vi "Configure Pattern Source.vi"(0 "VISA resource name":refnum<visa-resource-name>, 1 "Lower Threshold (1)":dbl, 2 "Data Mode (1: Fixed)":i32(ring) items=["Automatic", "Fixed"], 5 "Pattern Source (0: Internal)":i32(ring) items=["Internal", "External"], 7 "Voltage Range (5)":dbl, 9 "Impedance (1: 10000 Ohm)":i32(ring) items=["50 Ohm", "10000 Ohm"], 11 "error in (no error)":errorcluster, 12 "Upper Threshold (1.6)":dbl) -> (4 "VISA resource name out":refnum<visa-resource-name>, 15 "error out":errorcluster)   [LabVIEW 2009, in "Agilent 81150.lvlib"]
doc: "Configures the pattern source."
uses:
  Agilent 81150.lvlib
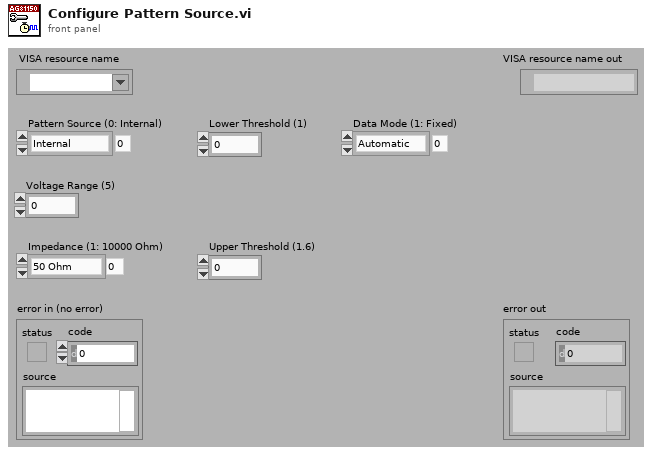
[diagram p1: front panel]
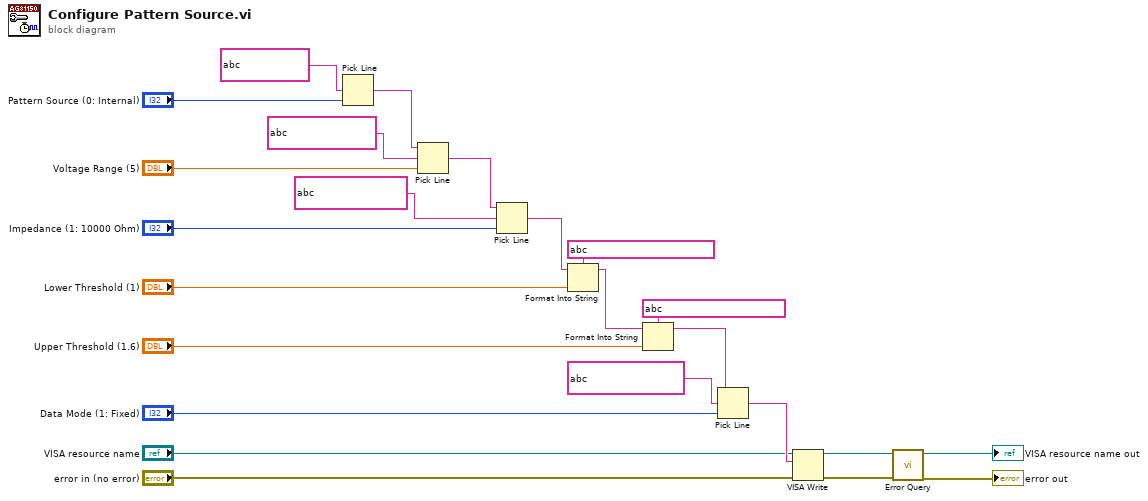
[diagram p0: block diagram]
diagram:
  n1 = Pick Line(multi-line string=string ?, line index="Pattern Source (0: Internal)") -> (output string=w20:string)  [unwired: 1 in]
  n2 = Pick Line(string ("")=w20, multi-line string=string ?, line index="Voltage Range (5)") -> (output string=w4:string)
  n3 = Pick Line(string ("")=w4, multi-line string=string ?, line index="Impedance (1: 10000 Ohm)") -> (output string=w1:string)
  n4 = Format Into String(format string=string ?, initial string=w1, "Lower Threshold (1)") -> (resulting string=w17:string)  [unwired: 1 in, 1 out]
  n5 = Format Into String(format string=string ?, initial string=w17, "Upper Threshold (1.6)") -> (resulting string=w12:string)  [unwired: 1 in, 1 out]
  n6 = Pick Line(string ("")=w12, multi-line string=string ?, line index="Data Mode (1: Fixed)") -> (output string=w11:string)
  n7 = VISA Write(VISA resource name="VISA resource name", write buffer=w11, error in (no error)="error in (no error)") -> (VISA resource name out=w8:refnum<visa-resource-name>, error out=w7:errorcluster)  [unwired: 1 out]
  n8 = call "Error Query.vi"("error in (no error)"=w7, "VISA resource name"=w8) -> ("error out"=→"error out":errorcluster, "VISA resource name out"=→"VISA resource name out":refnum<visa-resource-name>)  [unwired: 6 in, 2 out]
